vi "ORP_单点校准.vi"(7 "探头":u16(ring)=5 items=["NULL", "pH", "Cond", "DO", "Turb", "ORP", "6", "7", "COD", "9", "氯化物"], 8 "error in (no error)":errorcluster caption="错误输入（无错误）", 9 "信号值":sgl, 10 "标准值":sgl, 11 "MB session in":refnum<class "MB_Master.lvclass">) -> (0 "error out":errorcluster caption="错误输出", 3 "MB session out":refnum<class "MB_Master.lvclass">)   [LabVIEW 2022 SP3, in "斯坦道多参数.lvlib"]
uses:
  <vilib>/Plasmionique/MB Master/MB_Master/MB_Master.lvclass
  <vilib>/Plasmionique/MB Master/MB Master.lvlib
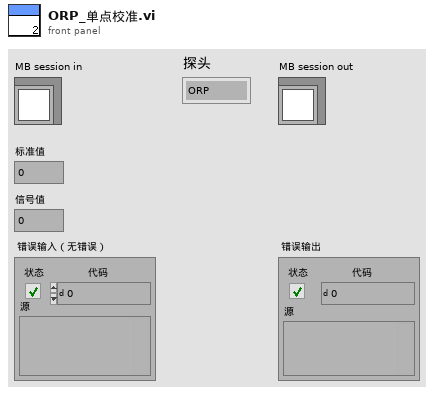
[diagram p1: front panel]
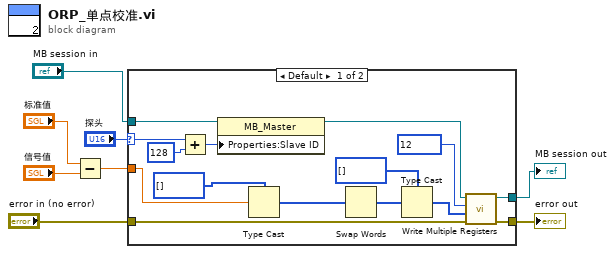
[diagram p0: block diagram]
diagram:
  n1 = Subtract(x="标准值", y="信号值") -> (x-y=w1:sgl)
  n2 = case shown="Default" "探头" {
    selector: "探头" -> [w9 _]
    tunnel: "error in (no error)" -> [w22 w24]
    tunnel: w1 -> [w14 _]
    tunnel: "MB session in" -> [w12 w25]
    tunnel: [w11 w24] -> w5
    tunnel: [w10 w25] -> w6
    frame Default {
      n3 = Add(x=w9, y=u16 128) -> (x+y=w21:u16)
      n4 = property class="MB_Master"(reference=w12, "Properties:Slave ID"=w21) -> (reference out=w19:refnum<class "MB_Master.lvclass">)  [unwired: 1 in, 1 out]
      n5 = Type Cast(type=u32[] [] ("数组 2"), x=w14) -> (*(type *) &x=w17:u32[])
      n6 = Swap Words(1:w17) -> (0:w15:u32[])
      n7 = Type Cast(type=u16[] [] ("数组 2"), x=w15) -> (*(type *) &x=w13:u16[])
      n8 = call <vilib>:"Write Multiple Registers.vi"("error in (no error)"=w22, "values"=w13, "starting address"=u16 12, "MB session in"=w19) -> ("error out"=w11:errorcluster, "MB session out"=w10:refnum<class "MB_Master.lvclass">)  [unwired: 6 in]
    }
    frame 0 {
    }
  }
  "error out" <- w5
  "MB session out" <- w6
